vi "Get Ring Exposure Range.vi"(10 "fpMax":sgl, 11 "fpMin":sgl) -> (1 "function return":u32, 2 "fpMax out":sgl, 3 "fpMin out":sgl)   [LabVIEW 2018, in "Copy of Andor SDK.lvlib"]
doc: "EXPNETTYPE unsigned int WINAPI GetRingExposureRange(float * fpMin, float * fpMax);"
uses:
  Copy of Andor SDK.lvlib
  <userlib>/Andor SDK/ATMCD32D.dll
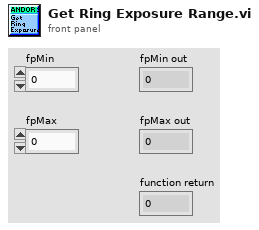
[diagram p1: front panel]
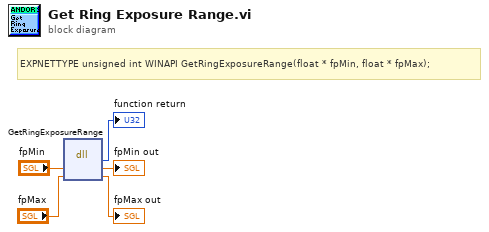
[diagram p0: block diagram]
diagram:
  # "EXPNETTYPE unsigned int WINAPI GetRingExposureRange(float * fpMin, float * fpMax);"
  n1 = dll-call lib="C:/Program Files (x86)/National Instruments/LabVIEW 2018/user.lib/Andor SDK/ATMCD32D.*" fn="GetRingExposureRange"("fpMin"="fpMin", "fpMax"="fpMax") -> (→"function return":u32, "fpMin"=→"fpMin out":sgl, "fpMax"=→"fpMax out":sgl)  [unwired: 3 in, 2 out]
